vi "AlternatingLEDs.vi"() -> ()   [LabVIEW 2014]
panel:
  in  "stop":bool
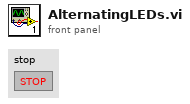
[diagram p1: front panel]
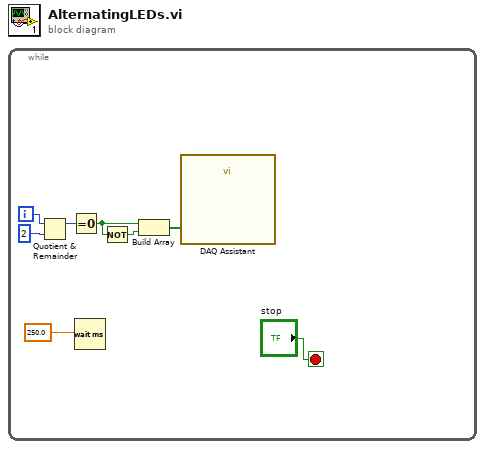
[diagram p0: block diagram]
diagram:
  n1 = while {
    i -> [w5]
    stop <- "stop" stop-if-true
    n2 = Quotient & Remainder(x=w5, y=2) -> (x-y*floor(x/y)=w3:i32)  [unwired: 1 out]
    n3 = Equal To 0?(x=w3) -> (x = 0?=w2:bool)
    n4 = Wait (ms)(milliseconds to wait=250.0) -> ()  [unwired: 1 out]
    n5 = Not(x=w2) -> (.not. x?=w7:bool)
    n6 = Build Array(w2, w7) -> (w8:bool[])
    n7 = call "DAQ Assistant"("data"=w8) -> ()  [unwired: 17 in, 2 out]
  }
